vi "Read (Multiple Points).vi"(8 "error in (no error)":errorcluster, 9 "Timeout (10000 ms)":i32=10000 format="%#.6g", 10 "Sample Count (1)":i32=1 min=1 max=50000, 11 "VISA resource name":refnum<visa-resource-name>) -> (0 "error out":errorcluster, 2 "Measurements":dbl[](array[numeric]), 3 "VISA resource name out":refnum<visa-resource-name>)   [LabVIEW 2020, in "PICOTEST M351XA Series.lvlib"]
doc: "Reads and returns multiple measurements from the instrument. Use this VI when you want to take multiple measurements using an immediate trigger. Use the low-level VIs for other triggering options."
uses:
  PICOTEST M351XA Series.lvlib
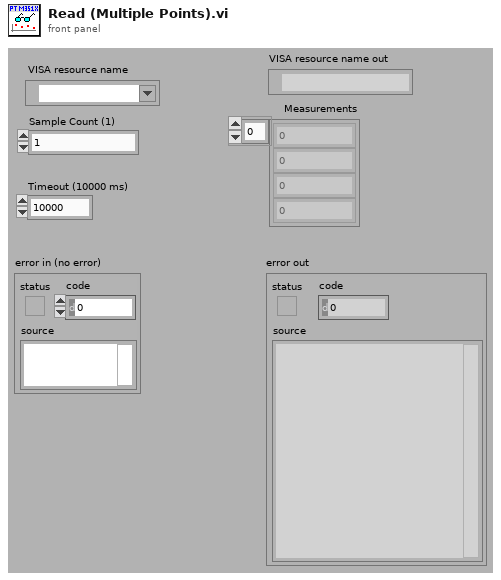
[diagram p1: front panel]
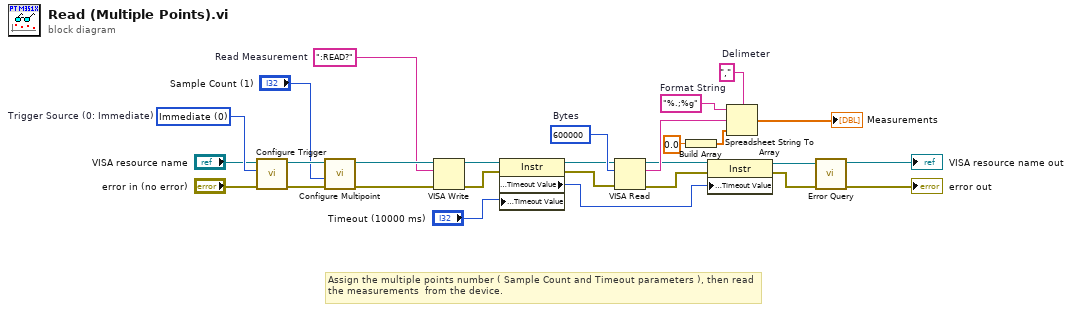
[diagram p0: block diagram]
diagram:
  w11 = u16 0 items=["Immediate", "Software (Bus)", "External"]  # Trigger Source (0: Immediate)
  w23 = ","  # Delimeter
  w24 = "%.;%g"  # Format String
  w3 = ":READ?"  # Read Measurement
  w28 = u32 600000  # Bytes
  # "Assign the multiple points number ( Sample Count and Timeout parameters ), then read the measurements  from the device."
  n1 = call "Configure Trigger.vi"("error in (no error)"="error in (no error)", "Trigger Source (0: Immediate)"=w11, "VISA resource name"="VISA resource name") -> ("error out"=w7:errorcluster, "VISA resource name out"=w8:refnum<visa-resource-name>)  [unwired: 7 in]
  n2 = call "Configure Multipoint.vi"("error in (no error)"=w7, "Sample Count (1)"="Sample Count (1)", "VISA resource name"=w8) -> ("error out"=w5:errorcluster, "VISA resource name out"=w4:refnum<visa-resource-name>)  [unwired: 7 in]
  n3 = VISA Write(VISA resource name=w4, write buffer=w3, error in (no error)=w5) -> (VISA resource name out=w2:refnum<visa-resource-name>, error out=w1:errorcluster)  [unwired: 1 out]
  n4 = property class="Instr"(reference=w2, error in=w1, "General Settings:Timeout Value"="Timeout (10000 ms)") -> (reference out=w19:refnum<visa-resource-name>, error out=w18:errorcluster, "General Settings:Timeout Value"=w12:u32)
  n5 = VISA Read(VISA resource name=w19, byte count=w28, error in (no error)=w18) -> (VISA resource name out=w16:refnum<visa-resource-name>, read buffer=w25:string, error out=w14:errorcluster)  [unwired: 1 out]
  n6 = Build Array(0.0) -> (w21:dbl[])
  n7 = property class="Instr"(reference=w16, error in=w14, "General Settings:Timeout Value"=w12) -> (reference out=w15:refnum<visa-resource-name>, error out=w13:errorcluster)
  n8 = Spreadsheet String To Array(delimiter (Tab)=w23, format string=w24, spreadsheet string=w25, array type (2D Dbl)=w21) -> (array=→"Measurements":dbl[])
  n9 = call "Error Query.vi"("error in (no error)"=w13, "VISA resource name"=w15) -> ("error out"=→"error out":errorcluster, "VISA resource name out"=→"VISA resource name out":refnum<visa-resource-name>)  [unwired: 6 in, 2 out]
